vi "SetFrameToCaptureNumber.vi"(8 "error in (no error)":errorcluster, 10 "Setting.FramesToCapture":i32, 11 "Camera_Prime95B in":refnum<class "Camera_Prime95B.lvclass">) -> (0 "error out":errorcluster, 3 "Camera_Prime95B out":refnum<class "Camera_Prime95B.lvclass">)   [LabVIEW 2020, in "Camera_Prime95B.lvlib" / "Camera_Prime95B.lvclass"]
uses:
  Camera_Prime95B.lvclass
  Camera_Prime95B.lvclass/Camera_Prime95B.ctl
  E:/Development/DevHardSoftware/MicroscopyFramework/Model/Hardware Layer/Real Hardware/Camera_Prime95B/Camera_Prime95B/Dependencies/PVCamNET.dll
  Dependencies/PVCamNET.dll
  Hardware Abstraction Layer/Component/Camera/Camera/Camera.lvclass
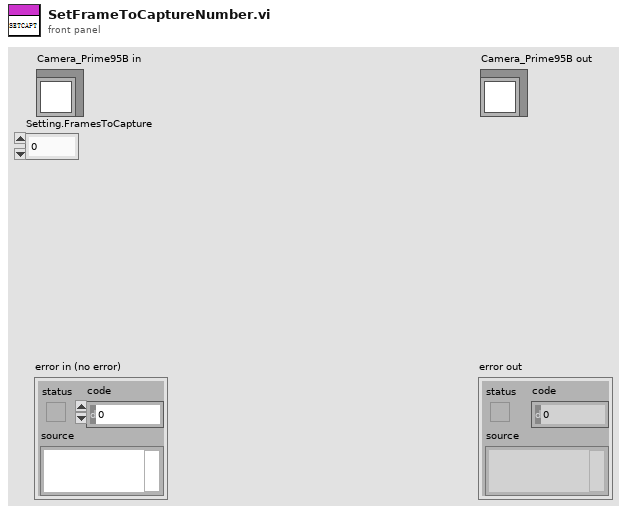
[diagram p1: front panel]
types:
  T1 = typedef "Device.lvlib/DeviceStatus.ctl" = i32
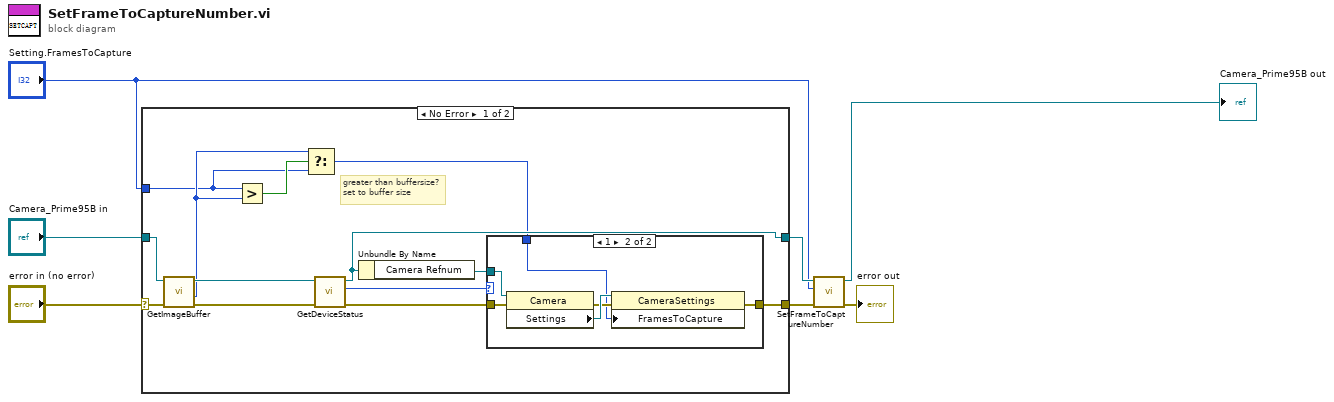
[diagram p0: block diagram]
diagram:
  n1 = case shown="No Error" "error in (no error)" {
    selector: "error in (no error)" -> [w19 w29]
    tunnel: [w20 w29] -> w4
    tunnel: "Camera_Prime95B in" -> [w13 w28]
    tunnel: [w15 w28] -> w3
    tunnel: "Setting.FramesToCapture" -> [w9 _]
    frame No Error {
      # "greater than buffersize?\nset to buffer size"
      n2 = call-dynamic "GetImageBuffer.vi"("error in (no error)"=w19, "Camera in"=w13) -> ("error out"=w14:errorcluster, "size(s)"=w10:i32, "Camera out"=w12:refnum<class "Camera_Prime95B.lvclass">)  [unwired: 6 in, 1 out]
      n3 = Greater?(x=w9, y=w10) -> (0:w11:bool)
      n4 = Select(t=w10, s=w11, f=w9) -> (s? t:f=w8:i32)
      n5 = call-dynamic "GetDeviceStatus.vi"("error in (no error)"=w14, "Camera_Prime95B in"=w12) -> ("error out"=w17:errorcluster, "Status"=w18:T1, "Camera_Prime95B out"=w15:refnum<class "Camera_Prime95B.lvclass">)  [unwired: 7 in]
      n6 = Unbundle By Name(w15) -> ("Camera Refnum"=w16:refnum<k24>)
      n7 = case shown="1" w18 {
        tunnel: [w21 w27] -> w20
        tunnel: w16 -> [_ w24]
        tunnel: w8 -> [_ w23]
        tunnel: w17 -> [w21 w22]
        frame 0, Default {
        }
        frame 1 {
          n8 = property class="Camera"(reference=w24, error in=w22) -> (error out=w25:errorcluster, "Settings"=w26:refnum<k24>)  [unwired: 1 out]
          n9 = property class="CameraSettings"(reference=w26, error in=w25, "FramesToCapture"=w23) -> (error out=w27:errorcluster)  [unwired: 1 out]
        }
      }
    }
    frame Error {
    }
  }
  n10 = call-parent "SetFrameToCaptureNumber.vi"("error in (no error)"=w4, "Setting.FramesToCapture"="Setting.FramesToCapture", "Camera in"=w3) -> ("error out"=→"error out":errorcluster, "Camera out"=→"Camera_Prime95B out":refnum<class "Camera_Prime95B.lvclass">)  [unwired: 7 in]
